vi "GUI.vi"() -> ()   [LabVIEW 2022 SP3]
uses:
  LABVIEW FILE'S/comman 2.o.vi
panel:
  out "Boolean 3":bool
  out "m":bool
  in  "String 3":string
  out "Tab Control 2":T1(tab)
  out "String":string
  out "Boolean 2":bool
  in  "Remove Button 2":bool
  out "Boolean":bool
  in  "Remove Button":bool
  in  "Blank Button 19":bool
  in  "OK Button":bool
  in  "Seek Back Button":bool
  in  "Cancel Button":bool
  in  "Blank Button 18":bool
  in  "Blank Button 17":bool
  in  "Blank Button 16":bool
  in  "Blank Button 15":bool
  in  "Blank Button 14":bool
  in  "Blank Button 13":bool
  in  "Blank Button 12":bool
  in  "Blank Button 11":bool
  in  "Blank Button 10":bool
  in  "Blank Button 9":bool
  in  "Blank Button 8":bool
  in  "Blank Button 7":bool
  in  "Blank Button 6":bool
  in  "Blank Button 5":bool
  in  "Blank Button 4":bool
  in  "Blank Button 3":bool
  in  "Blank Button 2":bool
  in  "Blank Button":bool
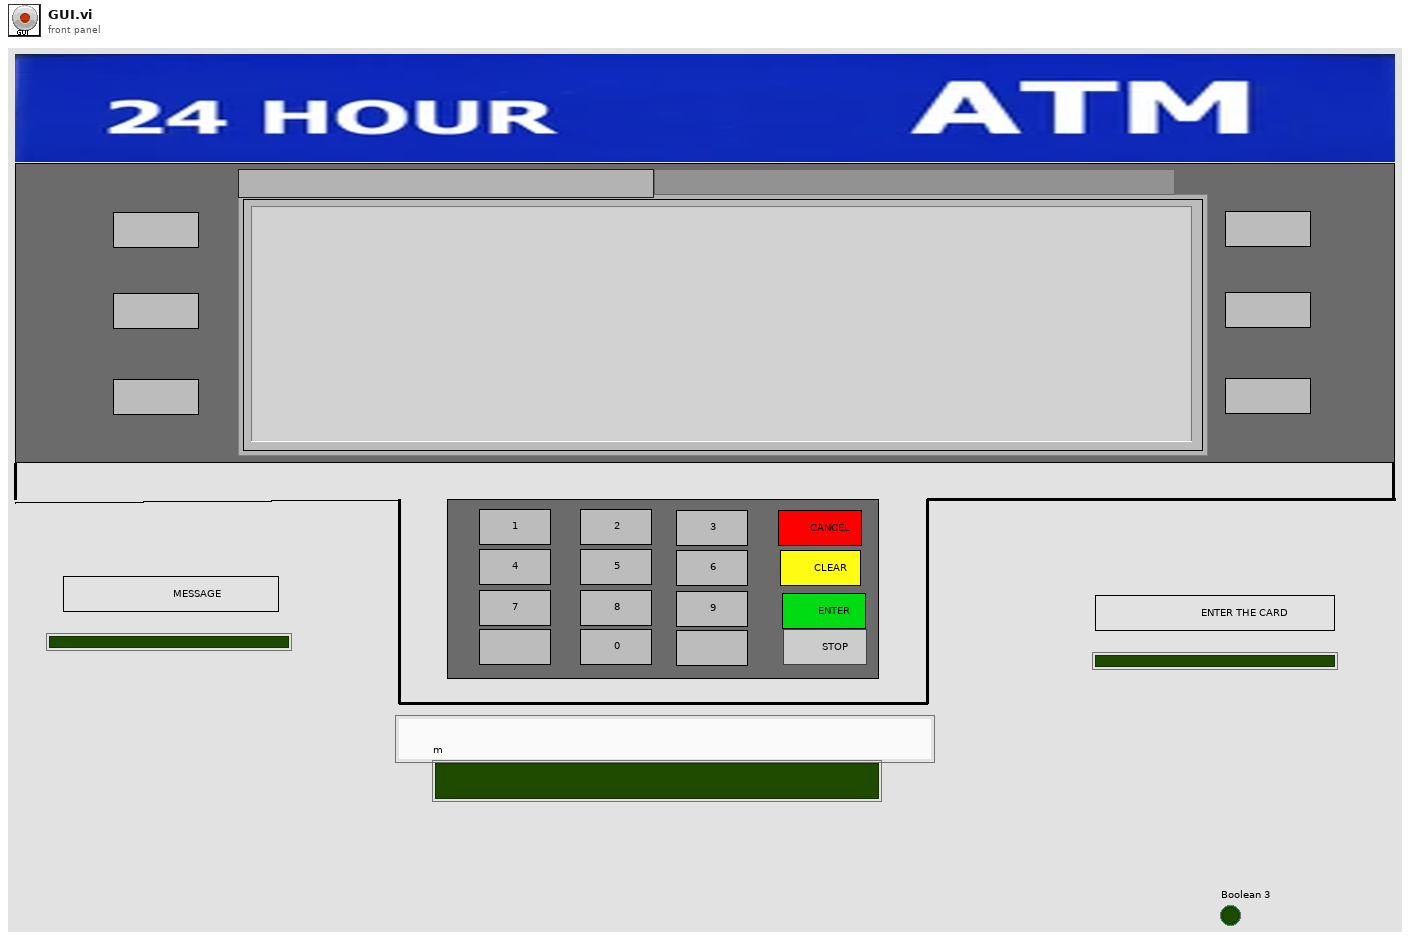
[diagram p1: front panel]
types:
  T1 = enum32{"                                                                                                                                      ", "                                                                                                                                                                         "}
  T2 = enum16{"ALL", "LANGUAGE", "MAIN MENU", "WITHDRAWALS", "BALANCE ENQUIRIES", "MINI STATEMENT", "CHANGE PIN", "FUND TRANSFER", "SERVICE", "english", "hindi", "tamil", "EVENT", "with1", "amount", "tran", "LED", "PIN", "mess", "welcome"}
  T3 = enum16{"ALL", "LANGUAGE", "MAIN MENU", "WITHDRAWALS", "BALANCE ENQUIRIES", "MINI STATEMENT", "CHANGE PIN", "FUND TRANSFER", "SERVICE", "english", "hindi", "tamil", "EVENT"}
  T4 = enum16{"ALL", "LANGUAGE", "MAIN MENU", "WITHDRAWALS", "BALANCE ENQUIRIES", "MINI STATEMENT", "CHANGE PIN", "FUND TRANSFER", "SERVICE", "english", "hindi", "tamil", "EVENT", "with1", "amount", "tran"}
  T5 = enum16{"ALL", "LANGUAGE", "MAIN MENU", "WITHDRAWALS", "BALANCE ENQUIRIES", "MINI STATEMENT", "CHANGE PIN", "FUND TRANSFER", "SERVICE", "english", "hindi", "tamil", "EVENT", "with1", "amount", "tran", "LED", "PIN", "mess"}
  T6 = enum16{"ALL", "LANGUAGE", "MAIN MENU", "WITHDRAWALS", "BALANCE ENQUIRIES", "MINI STATEMENT", "CHANGE PIN", "FUND TRANSFER", "SERVICE", "english", "hindi", "tamil", "EVENT", "with1", "amount", "tran", "LED", "PIN"}
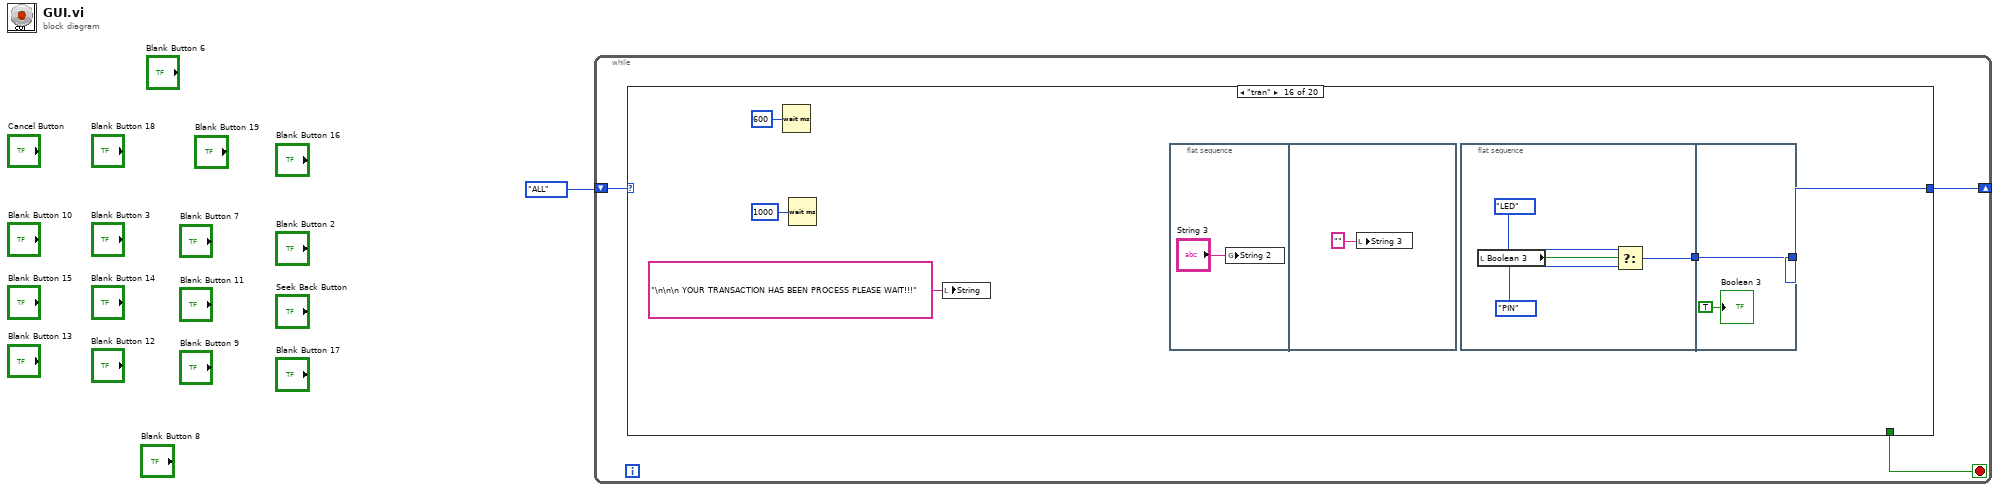
[diagram p0: block diagram]
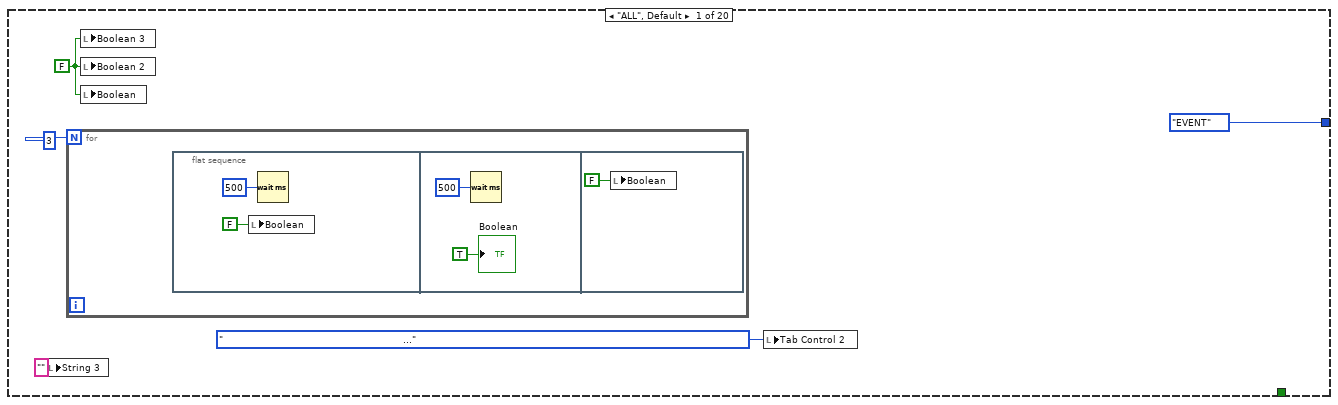
[diagram p2: hidden frame]
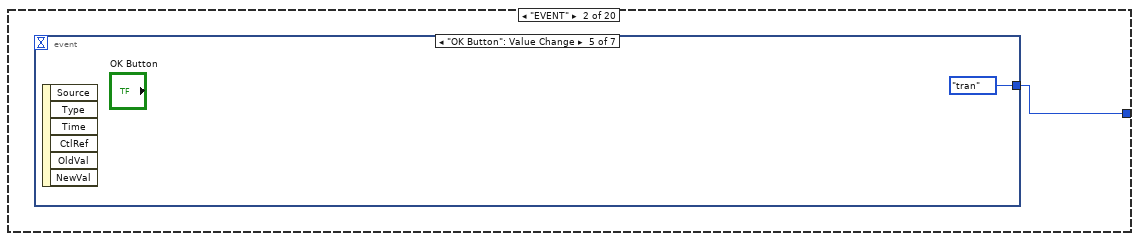
[diagram p3: hidden frame]
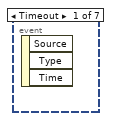
[diagram p4: hidden frame]
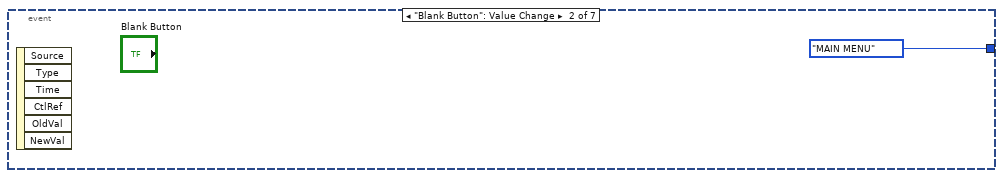
[diagram p5: hidden frame]
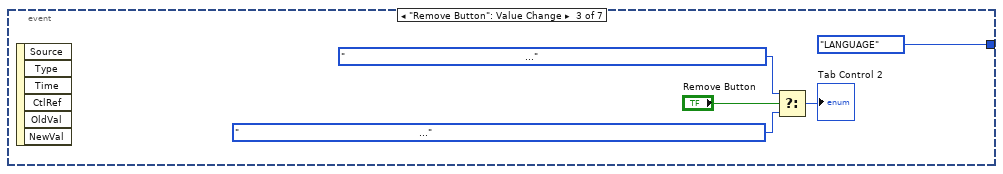
[diagram p6: hidden frame]
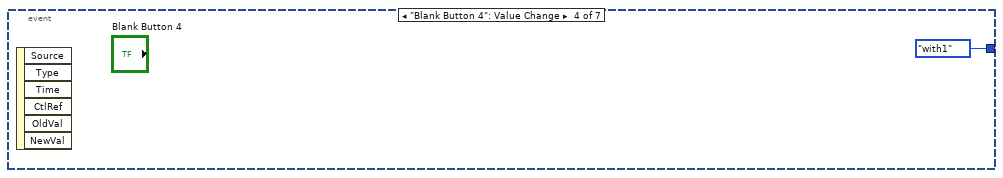
[diagram p7: hidden frame]
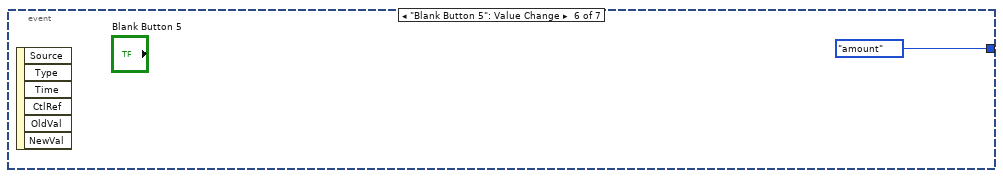
[diagram p8: hidden frame]
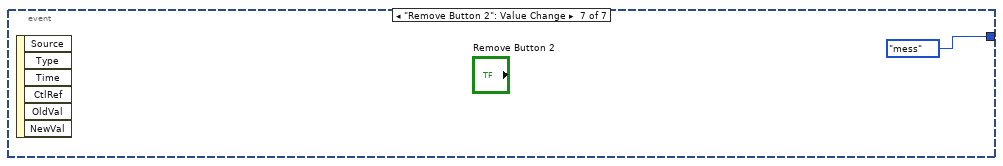
[diagram p9: hidden frame]
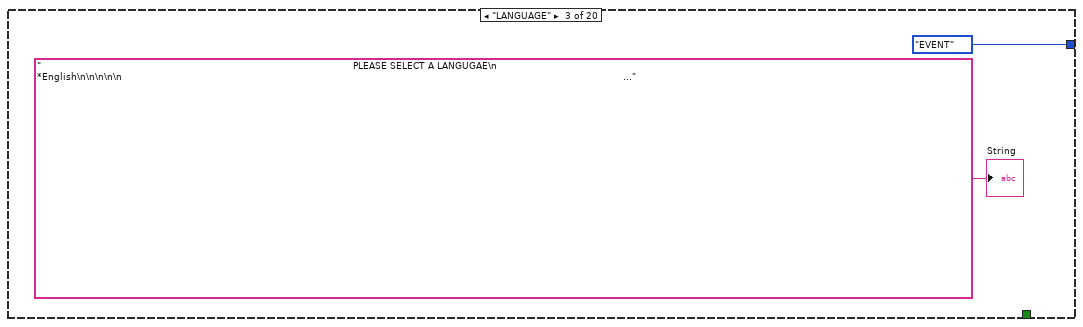
[diagram p10: hidden frame]
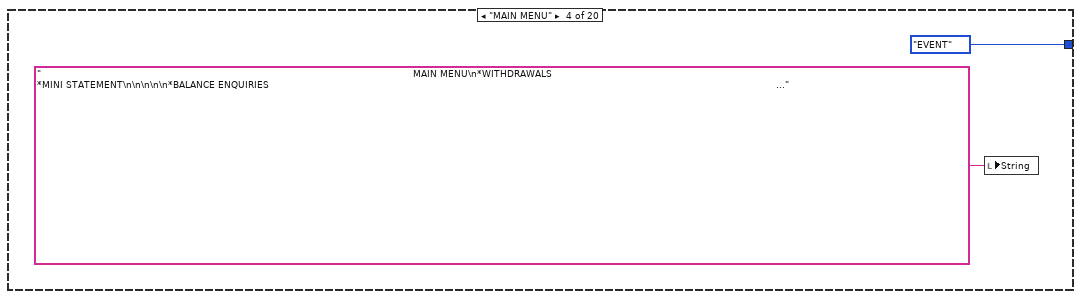
[diagram p11: hidden frame]
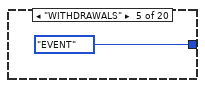
[diagram p12: hidden frame]
diagram:
  n1 = while {
    shift-right: [w4] -> _
    shift-left: T2."ALL" -> [w3]
    stop <- w2 stop-if-true
    n2 = case shown="\"tran\"" w3 {
      tunnel: [T3."EVENT" w15 T3."EVENT" T3."EVENT" T4."EVENT" _ _ _ _ _ _ _ _ T4."EVENT" T4."EVENT" w36 T5."EVENT" T2."welcome" T6."EVENT" _] -> w4
      tunnel: [_ _ _ _ _ _ _ _ _ _ _ _ _ _ _ _ _ FALSE ("Blank Button 19") _ TRUE ("Blank Button 19")] -> w2
      frame "ALL", Default {
        w5 = FALSE ("Boolean")
        n3 = local write "String 3"("") -> ()
        n4 = for {
          N: 3 -> [_]
          n5 = flat-sequence {
            frame #0 {
              n6 = local write "Boolean"(FALSE ("Boolean")) -> ()
              n7 = Wait (ms)(milliseconds to wait=u32 500) -> ()  [unwired: 1 out]
            }
            frame #1 {
              n8 = Wait (ms)(milliseconds to wait=u32 500) -> ()  [unwired: 1 out]
              "Boolean" <- TRUE ("Boolean")
            }
            frame #2 {
              n9 = local write "Boolean"(FALSE ("Boolean")) -> ()
            }
          }
        }
        n10 = local write "Boolean 3"(w5) -> ()
        n11 = local write "Boolean 2"(w5) -> ()
        n12 = local write "Boolean"(w5) -> ()
        n13 = local write "Tab Control 2"(T1."                                                                                                                                                                         " ("Tab Control 2")) -> ()
      }
      frame "EVENT" {
        n14 = event shown="[4] \"OK Button\": Value Change" {
          selector: _ -> [_ _ _ _ _ _ _]
          dyn-events: _ -> [_ _ _ _ _ _ _]
          timeout: _ -> [_ _ _ _ _ _ _]
          tunnel: [_ T3."MAIN MENU" T3."LANGUAGE" T4."with1" T4."tran" T4."amount" T5."mess"] -> w15
          event Timeout {
            n15 = event-data() -> ()  [unwired: 1 in, 3 out]
          }
          event "Blank Button": Value Change {
            n16 = event-data() -> ()  [unwired: 1 in, 6 out]
          }
          event "Remove Button": Value Change {
            n17 = event-data() -> ()  [unwired: 1 in, 6 out]
            n18 = Select(t=T1."                                                                                                                                      " ("Tab Control 2"), s="Remove Button", f=T1."                                                                                                                                                                         " ("Tab Control 2")) -> (s? t:f=→"Tab Control 2":T1)
          }
          event "Blank Button 4": Value Change {
            n19 = event-data() -> ()  [unwired: 1 in, 6 out]
          }
          event "OK Button": Value Change {
            n20 = event-data() -> ()  [unwired: 1 in, 6 out]
          }
          event "Blank Button 5": Value Change {
            n21 = event-data() -> ()  [unwired: 1 in, 6 out]
          }
          event "Remove Button 2": Value Change {
            n22 = event-data() -> ()  [unwired: 1 in, 6 out]
          }
        }
      }
      frame "LANGUAGE" {
        "String" <- "                                                                                                        PLEASE SELECT A LANGUGAE\n                                                                                                                                                                                                                                                                                                   *English\n\n\n\n\n                                                                                                                                                                                                                                                                                                    *Hindi\n\n\n\n\n\n                                                                                                                                                                                                                                                                                                    *Tamil                                                                                                                                                                                                                                                                                              "
      }
      frame "MAIN MENU" {
        n23 = local write "String"("                                                                                                                            MAIN MENU\n*WITHDRAWALS                                                                                                                                                                                                                                                       *MINI STATEMENT\n\n\n\n\n*BALANCE ENQUIRIES                                                                                                                                                                                                                                                *CHANGE PIN\n\n\n\n\n\n*FUND TRANSFER                                                                                                                                                                                                                                                        * SERVICE " ("String")) -> ()
      }
      frame "WITHDRAWALS" {
      }
      frame "BALANCE ENQUIRIES" {
      }
      frame "MINI STATEMENT" {
      }
      frame "CHANGE PIN" {
      }
      frame "FUND TRANSFER" {
      }
      frame "SERVICE" {
      }
      frame "tamil" {
      }
      frame "english" {
      }
      frame "hindi" {
      }
      frame "with1" {
        n24 = local write "String"("\n*CREAIT\n\n\n\n\n*SAVINGS\n\n\n\n\n\n*CURRENT" ("String")) -> ()
      }
      frame "amount" {
        n25 = local write "String"("                         \n\n\n\n\n\n                                                                                        PLEASE ENTER THE WITHDRAWAL AMOUNT IN MULTIPLES OF 500" ("String")) -> ()
      }
      frame "tran" {
        n26 = Wait (ms)(milliseconds to wait=u32 600) -> ()  [unwired: 1 out]
        n27 = Wait (ms)(milliseconds to wait=u32 1000) -> ()  [unwired: 1 out]
        n28 = local write "String"("\n\n\n YOUR TRANSACTION HAS BEEN PROCESS PLEASE WAIT!!!" ("String")) -> ()
        n29 = flat-sequence {
          frame #0 {
            n30 = global write "comman 2.o.vi" "String 2"("String 3") -> ()
          }
          frame #1 {
            n31 = local write "String 3"("" ("String 3")) -> ()
          }
        }
        n32 = flat-sequence {
          tunnel: [w43] -> w35
          tunnel: [w47] -> w36
          tunnel: w35 -> [w47]
          frame #0 {
            n33 = local read "Boolean 3"() -> (w42:bool)
            n34 = Select(t=T5."LED", s=w42, f=T5."PIN") -> (s? t:f=w43:T5)
          }
          frame #1 {
            "Boolean 3" <- TRUE ("Boolean 3")
          }
        }
      }
      frame "LED" {
        n35 = for {
          N: 3 -> [_]
          n36 = flat-sequence {
            frame #0 {
              n37 = local write "Boolean 2"(FALSE ("Boolean 2")) -> ()
              n38 = Wait (ms)(milliseconds to wait=u32 500) -> ()  [unwired: 1 out]
            }
            frame #1 {
              n39 = Wait (ms)(milliseconds to wait=u32 500) -> ()  [unwired: 1 out]
              "Boolean 2" <- TRUE ("Boolean 2")
            }
            frame #2 {
              n40 = local write "Boolean 2"(FALSE ("Boolean 2")) -> ()
              n41 = Wait (ms)(milliseconds to wait=u32 500) -> ()  [unwired: 1 out]
            }
          }
        }
      }
      frame "mess" {
        n42 = for {
          N: 5 -> [_]
          n43 = flat-sequence {
            frame #0 {
              n44 = local write "m"(FALSE ("m")) -> ()
              n45 = Wait (ms)(milliseconds to wait=u32 500) -> ()  [unwired: 1 out]
            }
            frame #1 {
              n46 = Wait (ms)(milliseconds to wait=u32 500) -> ()  [unwired: 1 out]
              "m" <- TRUE ("m")
            }
            frame #2 {
              n47 = Wait (ms)(milliseconds to wait=u32 500) -> ()  [unwired: 1 out]
              n48 = local write "m"(FALSE ("m")) -> ()
            }
          }
        }
        n49 = Concatenate Strings("message", ".vi" ("string")) -> (w59:string)
        n50 = call <vilib>:"Application Directory.vi"() -> ("Application Directory"=w66:path)
        n51 = Build Path(base path=w66, name or relative path=w59) -> (appended path=w65:path)
        n52 = Open VI Reference(vi path=w65) -> (vi reference=w64:refnum<vi>)  [unwired: 5 in, 1 out]
        n53 = invoke class="VI" method="FP.Open"(reference=w64) -> (reference out=w63:refnum<vi>, error out=w62:errorcluster)  [unwired: 4 in, 3 out]
        n54 = invoke class="VI" method="Run VI"(reference=w63, error in=w62) -> ()  [unwired: 3 in, 5 out]
      }
      frame "PIN" {
        n55 = local write "String"("                                     \n\n\n\n\n                                                                                                                  ENTER YOUR PIN NUMBER" ("String")) -> ()
      }
      frame "welcome" {
        n56 = flat-sequence {
          frame #0 {
            n57 = Wait (ms)(milliseconds to wait=u32 10000) -> ()  [unwired: 1 out]
            n58 = local write "String"("\n                                                                                                    PLEASE COLLECT YOUR CARD\n\n\n\n                                                                                                                             \"\"THANK YOU \"\"" ("String")) -> ()
          }
          frame #1 {
            n59 = local write "Tab Control 2"(T1."                                                                                                                                                                         " ("Tab Control 2")) -> ()
          }
        }
      }
    }
  }
